vi "下拉列表-按项名设置值.vi"(1 "项名":string, 2 "error in (no error)":errorcluster caption="错误输入（无错误）", 3 "下拉列表":refnum<vi>) -> (0 "error out":errorcluster caption="错误输出")   [LabVIEW 2014]
doc: "该模板用于创建子VI。"
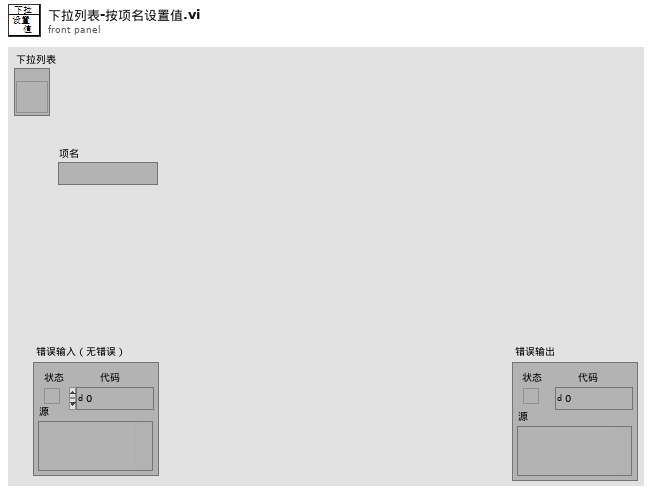
[diagram p1: front panel]
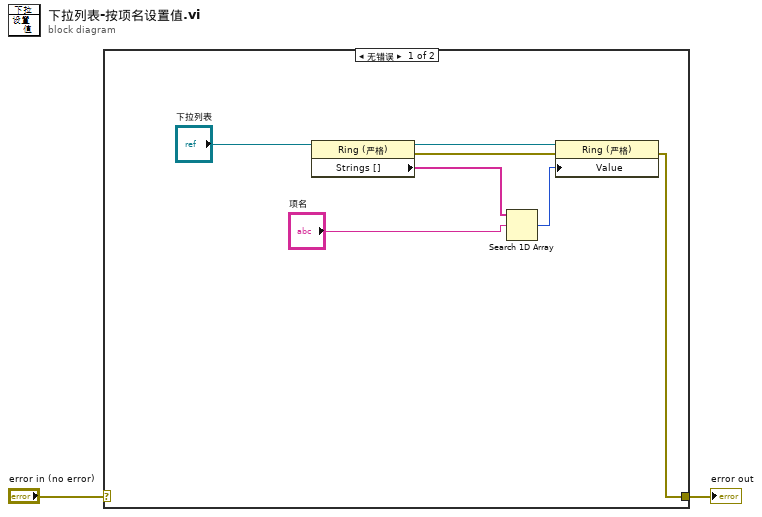
[diagram p0: block diagram]
diagram:
  n1 = case shown="无错误" "error in (no error)" {
    selector: "error in (no error)" -> [_ w10]
    tunnel: [w3 w10] -> w1
    frame No Error {
      n2 = property class="Ring (严格)"(reference="下拉列表") -> (reference out=w6:refnum<vi>, error out=w5:errorcluster, "Strings []"=w8:string[])  [unwired: 1 in]
      n3 = Search 1D Array(1D array=w8, element="项名") -> (index of element=w4:i32)  [unwired: 1 in]
      n4 = property class="Ring (严格)"(reference=w6, error in=w5, "Value"=w4) -> (error out=w3:errorcluster)  [unwired: 1 out]
    }
    frame Error {
    }
  }
  "error out" <- w1
